vi "RESETnumato board coomunication.vi"() -> ()   [LabVIEW 2018]
panel:
  in  "Command 3":string="reboot\r\n"
  out "read buffer 4":string
  out "read buffer":string
  out "read buffer 3":string
  in  "Command 2":string="admin\r\n"
  out "error out":errorcluster
  out "read buffer 2":string
  in  "Command":string="admin\r\n"
  in  "COM Port":refnum<visa-resource-name>
  # "TCPIP : : 192.168.1.100 : : 23 : : SOCKET"
  # "TCPIP0::192.168.1.100::23::SOCKET"
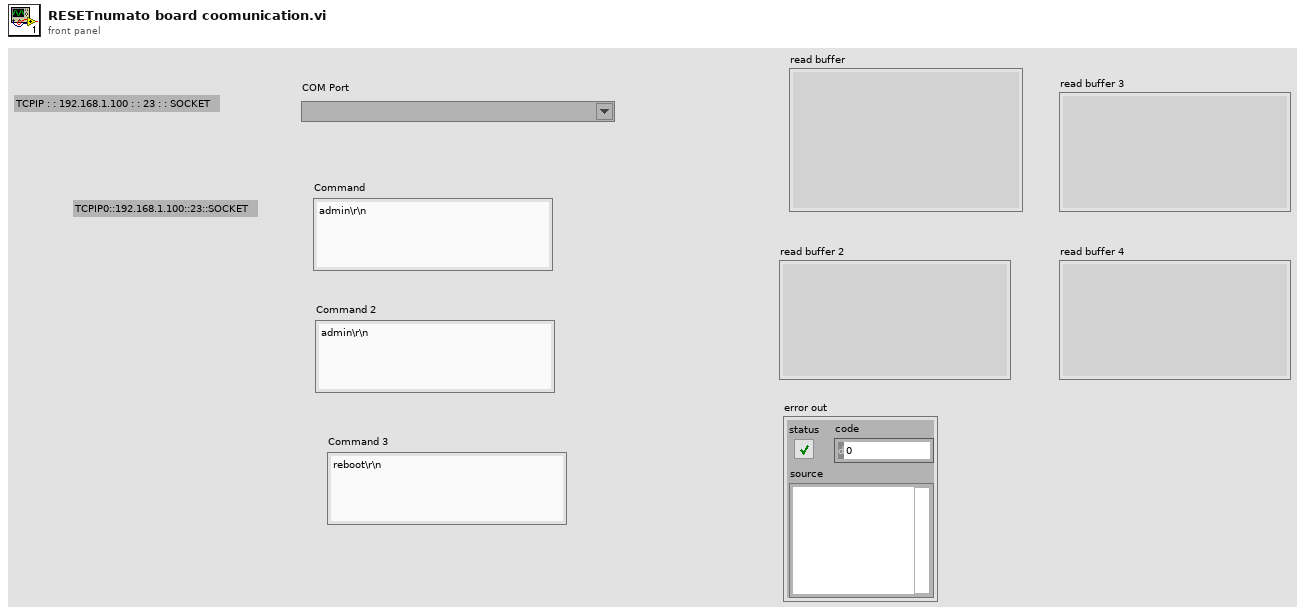
[diagram p1: front panel]
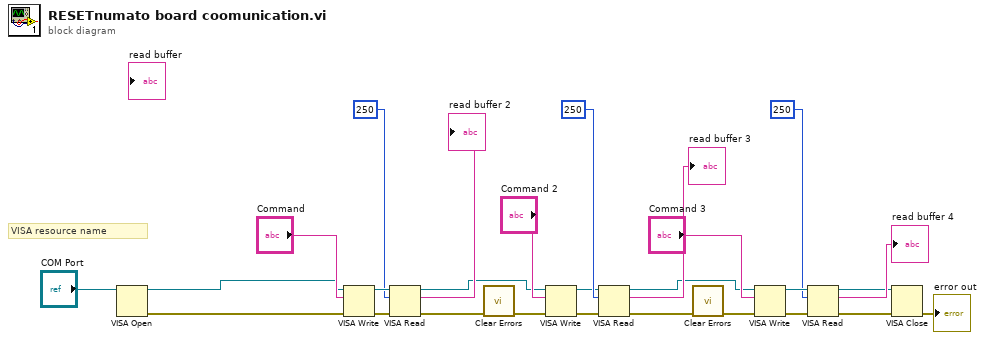
[diagram p0: block diagram]
diagram:
  # "VISA resource name"
  n1 = VISA Open(VISA resource name="COM Port") -> (VISA resource name=w2:refnum<visa-resource-name>, error out=w1:errorcluster)  [unwired: 4 in]
  n2 = VISA Write(VISA resource name=w2, write buffer="Command", error in (no error)=w1) -> (VISA resource name out=w26:refnum<visa-resource-name>, error out=w25:errorcluster)  [unwired: 1 out]
  n3 = VISA Read(VISA resource name=w26, byte count=u32 250, error in (no error)=w25) -> (VISA resource name out=w15:refnum<visa-resource-name>, read buffer=→"read buffer 2":string, error out=w14:errorcluster)  [unwired: 1 out]
  n4 = call <vilib>:"Clear Errors.vi"("error in (no error)"=w14) -> ("error out"=w13:errorcluster)  [unwired: 5 in, 1 out]
  n5 = VISA Write(VISA resource name=w15, write buffer="Command 2", error in (no error)=w13) -> (VISA resource name out=w17:refnum<visa-resource-name>, error out=w18:errorcluster)  [unwired: 1 out]
  n6 = VISA Read(VISA resource name=w17, byte count=u32 250, error in (no error)=w18) -> (VISA resource name out=w5:refnum<visa-resource-name>, read buffer=→"read buffer 3":string, error out=w6:errorcluster)  [unwired: 1 out]
  n7 = call <vilib>:"Clear Errors.vi"("error in (no error)"=w6) -> ("error out"=w12:errorcluster)  [unwired: 5 in, 1 out]
  n8 = VISA Write(VISA resource name=w5, write buffer="Command 3", error in (no error)=w12) -> (VISA resource name out=w10:refnum<visa-resource-name>, error out=w9:errorcluster)  [unwired: 1 out]
  n9 = VISA Read(VISA resource name=w10, byte count=u32 250, error in (no error)=w9) -> (VISA resource name out=w4:refnum<visa-resource-name>, read buffer=→"read buffer 4":string, error out=w3:errorcluster)  [unwired: 1 out]
  n10 = VISA Close(VISA resource name=w4, error in (no error)=w3) -> (error out=→"error out":errorcluster)
